vi "Start and End point of crosshair Y axis.vi"(10 "Crosshair":T1={"Draw"=TRUE, "Target"={"x"=20.0, "y"=20.0}, "Size"={"x"=20.0, "y"=20.0}, "Angle"=1250067.0, "Color"=1250067, "Thickness"=20, "CrosshairLabel"=""} {"Thickness" max=0; "Target"."y" min=0.0 max=0.0; "Target"."x" min=0.0 max=0.0; "Angle" format="%#_13g"; "Size"."y" min=0.0 max=0.0; "Size"."x" min=0.0 max=0.0}, 11 "Scaling factor":i32) -> (2 "Cluster 2":cluster{i32, i32}, 3 "Cluster":cluster{i32, i32})   [LabVIEW 2013]
uses:
  Controls/Crosshair type def.ctl
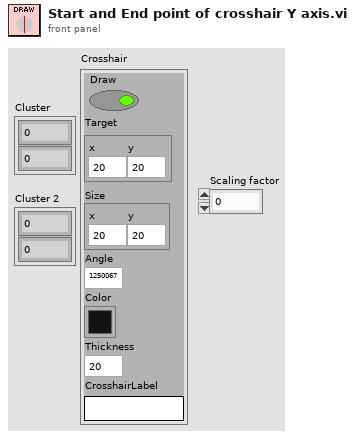
[diagram p1: front panel]
types:
  T1 = typedef "Crosshair type def.ctl" = cluster{"Draw":bool, "Target":cluster{"x":dbl, "y":dbl}, "Size":cluster{"x":dbl, "y":dbl}, "Angle":dbl, "Color":u32, "Thickness":u8, "CrosshairLabel":string}
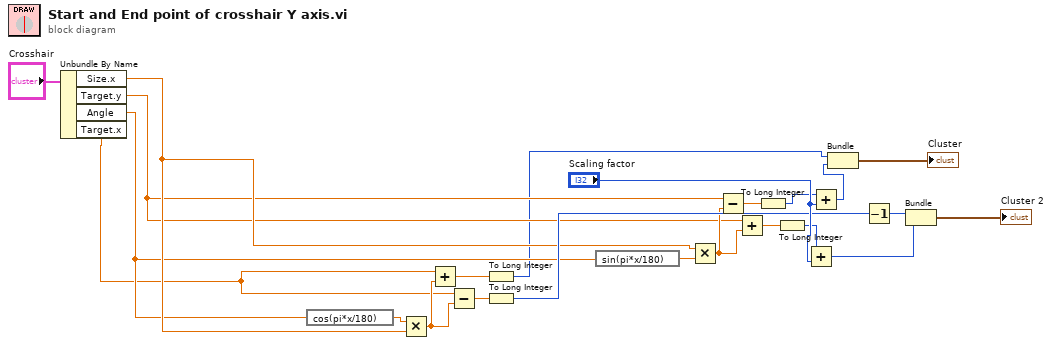
[diagram p0: block diagram]
diagram:
  n1 = Unbundle By Name("Crosshair") -> ("Size.x"=w7:dbl, "Target.y"=w6:dbl, "Angle"=w5:dbl, "Target.x"=w4:dbl)
  n2 = expression code="cos(pi*x/180)"(w5) -> (w15:dbl)
  n3 = Multiply(x=w15, y=w7) -> (x*y=w14:dbl)
  n4 = Add(x=w4, y=w14) -> (x+y=w16:dbl)
  n5 = Subtract(x=w4, y=w14) -> (x-y=w17:dbl)
  n6 = To Long Integer(number=w16) -> (32bit integer=w1:i32)
  n7 = To Long Integer(number=w17) -> (32bit integer=w20:i32)
  n8 = expression code="sin(pi*x/180)"(w5) -> (w12:dbl)
  n9 = Multiply(x=w7, y=w12) -> (x*y=w18:dbl)
  n10 = Subtract(x=w6, y=w18) -> (x-y=w13:dbl)
  n11 = Add(x=w6, y=w18) -> (x+y=w11:dbl)
  n12 = To Long Integer(number=w13) -> (32bit integer=w19:i32)
  n13 = To Long Integer(number=w11) -> (32bit integer=w21:i32)
  n14 = Add(x=w21, y="Scaling factor") -> (x+y=w23:i32)
  n15 = Add(x=w19, y="Scaling factor") -> (x+y=w3:i32)
  n16 = Bundle(w1, w3) -> (→"Cluster":cluster{i32, i32})  [unwired: 1 in]
  n17 = Decrement(x=w20) -> (x-1=w2:i32)
  n18 = Bundle(w2, w23) -> (→"Cluster 2":cluster{i32, i32})  [unwired: 1 in]
